vi "JLINKARM Read Mem.vi"(8 "error in (no error)":errorcluster caption="错误输入（无错误）", 9 "buff":string, 10 "size":u32, 11 "memaddr":u32) -> (0 "error out":errorcluster caption="错误输出", 1 "buff out":string, 3 "function return":i32)   [LabVIEW 2016, in "JLinkARM.lvlib"]
doc: "int JLINKARM_ReadMem(unsigned long memaddr,unsigned long size,unsigned char * buff);"
uses:
  <userlib>/LV-JLinkARM/JLinkARM.lvlib
  <userlib>/LV-JLinkARM/JLinkARM.dll
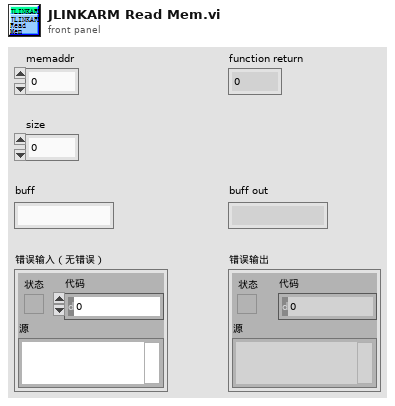
[diagram p1: front panel]
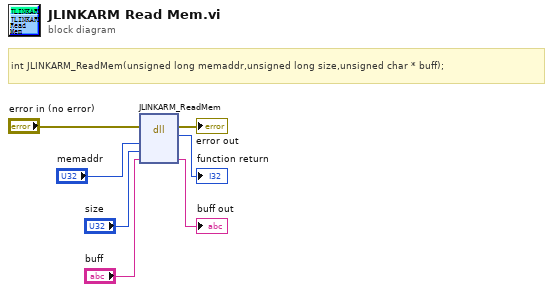
[diagram p0: block diagram]
diagram:
  # "int JLINKARM_ReadMem(unsigned long memaddr,unsigned long size,unsigned char * buff);"
  n1 = dll-call lib="C:/Program Files (x86)/National Instruments/LabVIEW 2016/user.lib/LV-JLinkARM/JLinkARM.*" fn="JLINKARM_ReadMem"(error in="error in (no error)", "memaddr"="memaddr", "size"="size", "buff"="buff") -> (error out=→"error out":errorcluster, →"function return":i32, "buff"=→"buff out":string)  [unwired: 4 in, 1 out]
